vi "Read Index and SubIndex.vi"(8 "error in (no error)":errorcluster, 10 "Section":string, 11 "Clust Refnum":refnum<vi>) -> (0 "error out":errorcluster, 3 "dup Clust Refnum":refnum<vi>)   [LabVIEW 2013]
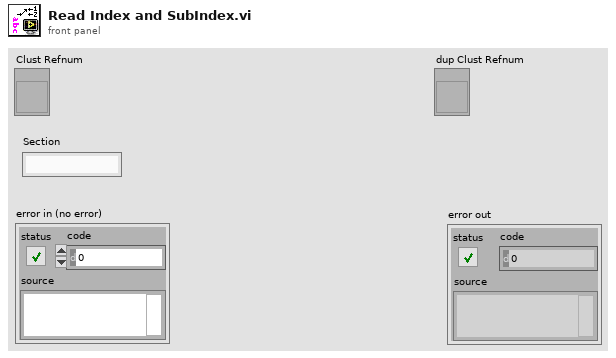
[diagram p1: front panel]
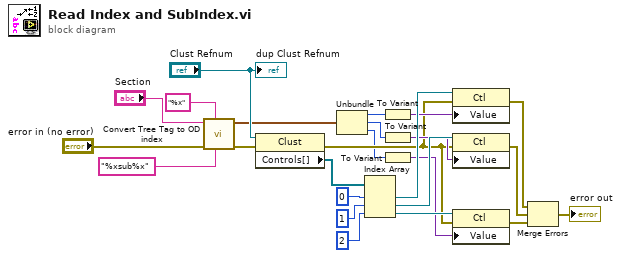
[diagram p0: block diagram]
diagram:
  n1 = call "Convert Tree Tag to OD index.vi"("subindex format"="%xsub%x" ("format string"), "index format"="%x" ("format string"), "error in"="error in (no error)", "Tag"="Section") -> ("error out"=w8:errorcluster, "index"=w4:cluster{u16, u8, u8})  [unwired: 6 in]
  n2 = property class="Clust"(reference="Clust Refnum", error in=w8) -> (error out=w12:errorcluster, "Controls[]"=w25:refnum<vi>[])  [unwired: 1 out]
  n3 = Unbundle(w4) -> (w3:u16, w2:u8, w1:u8)
  n4 = Index Array(array=w25, index #1=0 ("index"), index #2=1 ("index"), index #3=2 ("index")) -> (element #1=w22:refnum<vi>, element #2=w21:refnum<vi>, element #3=w13:refnum<vi>)
  n5 = To Variant(anything=w3) -> (Variant=w20:variant)
  n6 = To Variant(anything=w2) -> (Variant=w19:variant)
  n7 = To Variant(anything=w1) -> (Variant=w11:variant)
  n8 = property class="Ctl"(reference=w22, error in=w12, "Value"=w20) -> (error out=w18:errorcluster)  [unwired: 1 out]
  n9 = property class="Ctl"(reference=w21, error in=w12, "Value"=w19) -> (error out=w17:errorcluster)  [unwired: 1 out]
  n10 = property class="Ctl"(reference=w13, error in=w12, "Value"=w11) -> (error out=w10:errorcluster)  [unwired: 1 out]
  n11 = Merge Errors(w18, w17, w10) -> (→"error out":errorcluster)
  "dup Clust Refnum" <- "Clust Refnum"
